vi "Configure Power Sensor Resolution.vi"(8 "error in (no error)":errorcluster, 9 "Resolution (0.01 dB)":i32(ring)=2 items=["1 dB", "0.1 dB", "0.01 dB", "0.001 dB"], 10 "Instance (1)":i32=1 format="%.0g", 11 "VISA resource name":refnum<visa-resource-name>) -> (0 "error out":errorcluster, 3 "VISA resource name out":refnum<visa-resource-name>)   [LabVIEW 2015, in "Rohde&Schwarz CMXP GPRF.lvlib"]
doc: "Defines the number of digits of the power results in the measurement dialog. This command does not affect the remote control results.\n\nAttribute:\nRSCMXPGPRF_ATTR_SENSOR_MEASUREMENT_RESOLUTION\n\nRemote-control command:\nCONFigure:GPRF:MEAS<i>:EPSensor:RESolution"
uses:
  <instrlib>/Rohde&Schwarz CMXP GPRF/Rohde&Schwarz CMXP GPRF.lvlib
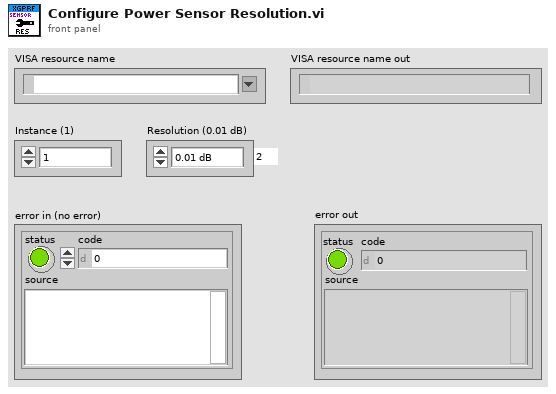
[diagram p1: front panel]
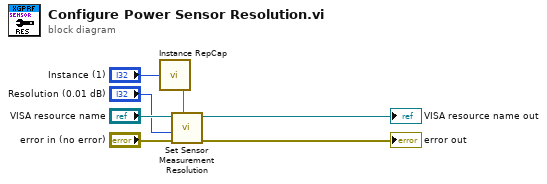
[diagram p0: block diagram]
diagram:
  n1 = call <instrlib>:"Instance RepCap.vi"("instance  in"="Instance (1)") -> ("instance out"=w4:string)
  n2 = call "Set Sensor Measurement Resolution"("Repeated Capabilities"=w4, "error in (no error)"="error in (no error)", "Sensor Measurement Resolution (0 - 1 dB)"="Resolution (0.01 dB)", "instrument handle"="VISA resource name") -> ("error out"=→"error out":errorcluster, "instrument handle out"=→"VISA resource name out":refnum<visa-resource-name>)  [unwired: 6 in]
